vi "PmacFileDownLoad.vi"(2 "Down Load File Path":path, 3 "Device Number i32 (0)":i32 min=0) -> (0 "Down Load Log File Path":path, 1 "Down Load Error Bool (F)":bool)   [LabVIEW 2020]
doc: "Compile the ASCII motion or PLC program specified by Down Load File Path and down load the compiled code to PMAC. If there is a compile error Down Load Error is TRUE. Down Load Log File Path specifies the path to the compile log file. \n\nExample\n\nIf Down Load File Path is PmacTest1.pmc this path is PmacTest1.log. If there is a compile error a pop-up panel displaying the log file appears to detail compile and down load errors."
uses:
  Builds/5-8-13/data/PComm32W.dll
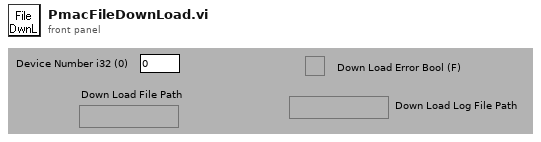
[diagram p1: front panel]
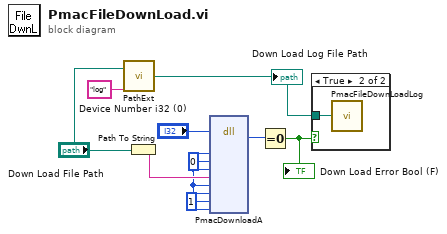
[diagram p0: block diagram]
diagram:
  w8 = 1
  w6 = 0
  n1 = call "PathExt.vi"("New Extension"="log", "Down Load File Path"="Down Load File Path") -> ("Down Load Log File Path"=w2:path)
  "Down Load Log File Path" <- w2
  n2 = Path To String(path="Down Load File Path") -> (string=w7:string)
  n3 = dll-call lib="C:/NUWAR_Master/Builds/5-8-13/data/PComm32W.dll" fn="PmacDownloadA" label="PmacDownloadFile"("DeviceNumber"="Device Number i32 (0)", "msgp"=w6, "getp"=w6, "pprg"=w6, "FileName"=w7, "macro"=w6, "map"=w6, "log"=w8, "dnld"=w8) -> (w9:i32)  [unwired: 12 in, 2 out]
  n4 = Equal To 0?(x=w9) -> (x = 0?=w1:bool)
  "Down Load Error Bool (F)" <- w1
  n5 = case shown="True" w1 {
    tunnel: w2 -> [_ w10]
    frame False {
    }
    frame True {
      n6 = call "PmacFileDownLoadLog.vi"("Log File Path"=w10) -> ()
    }
  }
